vi "Autorunner.vi"() -> ()   [LabVIEW 2017, in "Fridge Software v2.1.lvlib"]
uses:
  Fridge Software v2.1.lvlib
  <vilib>/Platform/TimedLoop/XDataNode/timing_clust.ctl
  <vilib>/Platform/TimedLoop/XDataNode/nitl_modes.ctl
  <vilib>/Platform/TimedLoop/XDataNode/wakeup.ctl
  <vilib>/Utility/file.llb/Read Delimited Spreadsheet (DBL).vi
  <vilib>/Utility/file.llb/Read Delimited Spreadsheet (string).vi
  <vilib>/Utility/file.llb/Write Delimited Spreadsheet (DBL).vi
  <vilib>/platform/TimedLoop/XDataNode/XDataNode.xnode
  <instrlib>/Lake Shore 372/Lake Shore 372.lvlib
  <instrlib>/Keithley 3706/Keithley 3700 Series.lvlib
  <vilib>/Platform/TimedLoop/XDataNode/XDNodeRunTimeDep.lvlib
panel:
  in  "R(T,H) tab":enum32{"R(T)", "R(H)"}(tab)
  in  "Clear R(T) graph":bool
  in  "Autoscale R(T)":bool=TRUE caption="Autoscale"
  out "R(T) Graph":cluster{dbl[], dbl[]}(graph)
  in  "Clear H(T) graph":bool
  in  "Autoscale H(T)":bool=TRUE caption="Autoscale"
  out "R(H) Graph":cluster{dbl[], dbl[]}(graph)
  in  "Clear H(t) graph":bool
  in  "Clear T(t) graph":bool
  in  "Clear R(t) graph":bool
  in  "Autoscale H(t)":bool=TRUE caption="Autoscale"
  in  "Autoscale T(t)":bool=TRUE caption="Autoscale"
  in  "Autoscale R(t)":bool=TRUE caption="Autoscale"
  out "H(t) Graph 4":cluster{dbl[], dbl[]}(graph)
  out "T(t) Graph 3":cluster{dbl[], dbl[]}(graph)
  out "R(t) Graph":cluster{dbl[], dbl[]}(graph)
  out "Input Reading Status Query":string
  out "Elapsed time":dbl=500.0 min=50.0 step=100.0
  out "Magnetic Poles \nLive  Voltage":dbl format="%#_5g"
  in  "Measurement\nperiod":i64=500 min=100 step=100
  out "Power Reading":dbl min=0.0 max=0.01 step=1e-05 format="%^.3g"
  out "Sample Reactance":dbl min=0.0 max=63200000.0 step=1e-05 format="%.3g"
  out "Cernox Resistance":dbl min=0.0 max=63200000.0 step=1e-05 format="%.3g"
  out "Sample Resistance":dbl min=0.0 max=63200000.0 step=1e-05 format="%^.5g"
  out "Cernox Temperature":dbl min=0.0 max=1000.0 step=1e-05 format="%.4f"
  in  "Measurement":T1(tab)
  in  "Hall probe/Aux":bool
  in  "Lakeshore port":refnum<visa-resource-name>="COM6"
  in  "Cernox Channel":u16(ring)=17 caption="Cernox" items=["1"=1, "2"=2, "3"=3, "4"=4, "5"=5, "6"=6, "7"=7, "8"=8, "9"=9, "10"=10, "11"=11, "12"=12, "13"=13, "14"=14, "15"=15, "16"=16, "A"=17]
  in  "Sample Channel":u16(ring)=1 caption="Sample" items=["1"=1, "2"=2, "3"=3, "4"=4, "5"=5, "6"=6, "7"=7, "8"=8, "9"=9, "10"=10, "11"=11, "12"=12, "13"=13, "14"=14, "15"=15, "16"=16, "A (Control Input)"=17]
  in  "Switchboard port":refnum<visa-resource-name>="USB0::0x05E6::0x3706::04089883::INSTR"
  in  "Arduino port \n(for magnetic poles)":refnum<visa-resource-name>="COM3"
  out "Lakeshore Error":errorcluster
  in  "Update":bool
  out "Excitation  Ind":bool=TRUE
  out "Excitation Mode Ind":u16(ring)=1 items=["Voltage", "Current"]
  out "Excitation Range Ind":u16(ring)=19 items=["31.6 mA"=22, "10.0 mA"=21, "3.16 mA"=20, "1.00 mA"=19, "316 uA"=18, "100 uA"=17, "31.6 uA"=16, "10.0 uA"=15, "3.16 uA"=14, "1.00 uA"=13, "632 mV / 316 nA"=12, "200 mV / 100 nA"=11, "63.2 mV / 31.6 nA"=10, "20.0 mV / 10.0 nA"=9, "6.32 mV / 3.16 nA"=8, "2.00 mV / 1.00 nA"=7, "632 uV / 316 pA"=6, "200 uV / 100 pA"=5, "63.2 uV / 31.6 pA"=4, "20.0 uV / 10.0 pA"=3, "6.32 uV / 3.16 pA"=2, "2.00 uV / 1.00 pA"=1]
  out "Autorange Ind":u16(ring) items=["Autorange off", "Autorange Current", "ROX 102B Autorange"]
  out "Resistance Range Ind":u16(ring)=8 items=["63.2 MOhm"=22, "20.0 MOhm"=21, "6.32 MOhm"=20, "2.00 MOhm"=19, "632 kOhm"=18, "200 kOhm"=17, "63.2 kOhm"=16, "20.0 kOhm"=15, "6.32 kOhm"=14, "2.00 kOhm"=13, "632 Ohm"=12, "200 Ohm"=11, "63.2 Ohm"=10, "20.0 Ohm"=9, "6.32 Ohm"=8, "2.00 Ohm"=7, "632 mOhm"=6, "200 mOhm"=5, "63.2 mOhm"=4, "20.0 mOhm"=3, "6.32 mOhm"=2, "2.00 mOhm"=1]
  out "Preferred Units Ind":u16(ring)=2 items=["Kelvin"=1, "Ohms"=2]
  out "Temperature Limit Ind":dbl min=0.0 max=2999.0 step=1.0
  in  "Excitation Mode":u16(ring)=1 items=["Voltage", "Current"]
  in  "Excitation Range":u16(ring)=19 items=["31.6 mA"=22, "10.0 mA"=21, "3.16 mA"=20, "1.00 mA"=19, "316 uA"=18, "100 uA"=17, "31.6 uA"=16, "10.0 uA"=15, "3.16 uA"=14, "1.00 uA"=13, "632 mV / 316 nA"=12, "200 mV / 100 nA"=11, "63.2 mV / 31.6 nA"=10, "20.0 mV / 10.0 nA"=9, "6.32 mV / 3.16 nA"=8, "2.00 mV / 1.00 nA"=7, "632 uV / 316 pA"=6, "200 uV / 100 pA"=5, "63.2 uV / 31.6 pA"=4, "20.0 uV / 10.0 pA"=3, "6.32 uV / 3.16 pA"=2, "2.00 uV / 1.00 pA"=1]
  in  "Autorange (0: Autorange off)":u16(ring) items=["Autorange off", "Autorange Current", "ROX 102B Autorange"]
  in  "Resistance Range":u16(ring)=8 items=["63.2 MOhm"=22, "20.0 MOhm"=21, "6.32 MOhm"=20, "2.00 MOhm"=19, "632 kOhm"=18, "200 kOhm"=17, "63.2 kOhm"=16, "20.0 kOhm"=15, "6.32 kOhm"=14, "2.00 kOhm"=13, "632 Ohm"=12, "200 Ohm"=11, "63.2 Ohm"=10, "20.0 Ohm"=9, "6.32 Ohm"=8, "2.00 Ohm"=7, "632 mOhm"=6, "200 mOhm"=5, "63.2 mOhm"=4, "20.0 mOhm"=3, "6.32 mOhm"=2, "2.00 mOhm"=1]
  in  "Preferred Units (2: Ohms)":u16(ring)=2 items=["Kelvin"=1, "Ohms"=2]
  in  "Temperature Limit (0 Kelvin)":dbl min=0.0 max=2999.0 step=1.0
  in  "Excitation  (T: On)":bool=TRUE caption="On\n\nOff"
  in  "Grab settings":bool
  out "Heater Output Ind":dbl
  out "Heater Setpoint":dbl
  out "Heater Setpoint Ind":dbl
  in  "Grab Heater settings":bool
  in  "Update Heater Settings":bool
  in  "I+":i32 min=0 max=24 step=1
  in  "I-":i32 min=0 max=24 step=1
  in  "V+":i32 min=0 max=24 step=1
  in  "V-":i32 min=0 max=24 step=1
  in  "Close pins (safe)":bool caption="Close I-V pins -> Lift ground -> Lift common -> Current on"
  in  "Lift pins (safe)":bool caption="Current off -> Common closed -> Ground -> Lift I-V pins"
  in  "Channel Open/Close Array":string
  in  "Open":bool
  in  "Close":bool
  in  "Open All IV":bool
  out "Closed Channels":string
  out "Ground closed":bool
  out "Common rail \nclosed":bool
  out "Common-ground \nlink closed":bool
  in  "Append file":bool
  in  "File path":path
  in  "Save Data":bool
  in  "Aux max voltage (mV)":dbl
  in  "Aux Field Range (Oe)":dbl
  in  "Skip temperature checker":bool
  in  "Data Acquisition time\n(mins)":dbl
  in  "T Array File":path
  in  "Device/Pin Array File":path
  # "Autorunner"
  # "Created by Daniel Bromley & Alex Wright, IPF Ltd 2021"
  # "s"
  # "V"
  # "ms"
  # "W"
  # "jW"
  # "W"
  # "W"
  # "K"
  # "Lakeshore - Measurement"
  # "Channels:"
  # "Keithley - Switchboard"
  # "Hall probe"
  # "Aux"
  # "Lakeshore setting"
  # "User setting"
  # "Excitation Mode"
  # "Excitation Range"
  # "Autorange"
  # "Resistance Range"
  # "Preferred Units"
  # "Temperature Limit"
  # "Excitation"
  # "Lakeshore setting"
  # "User setting"
  # "Heater Setpoint"
  # "Heater output"
  # "IV pins"
  # "Array"
  # "Set Filename and Path"
  # "(Will be appended by Device name and temperature)"
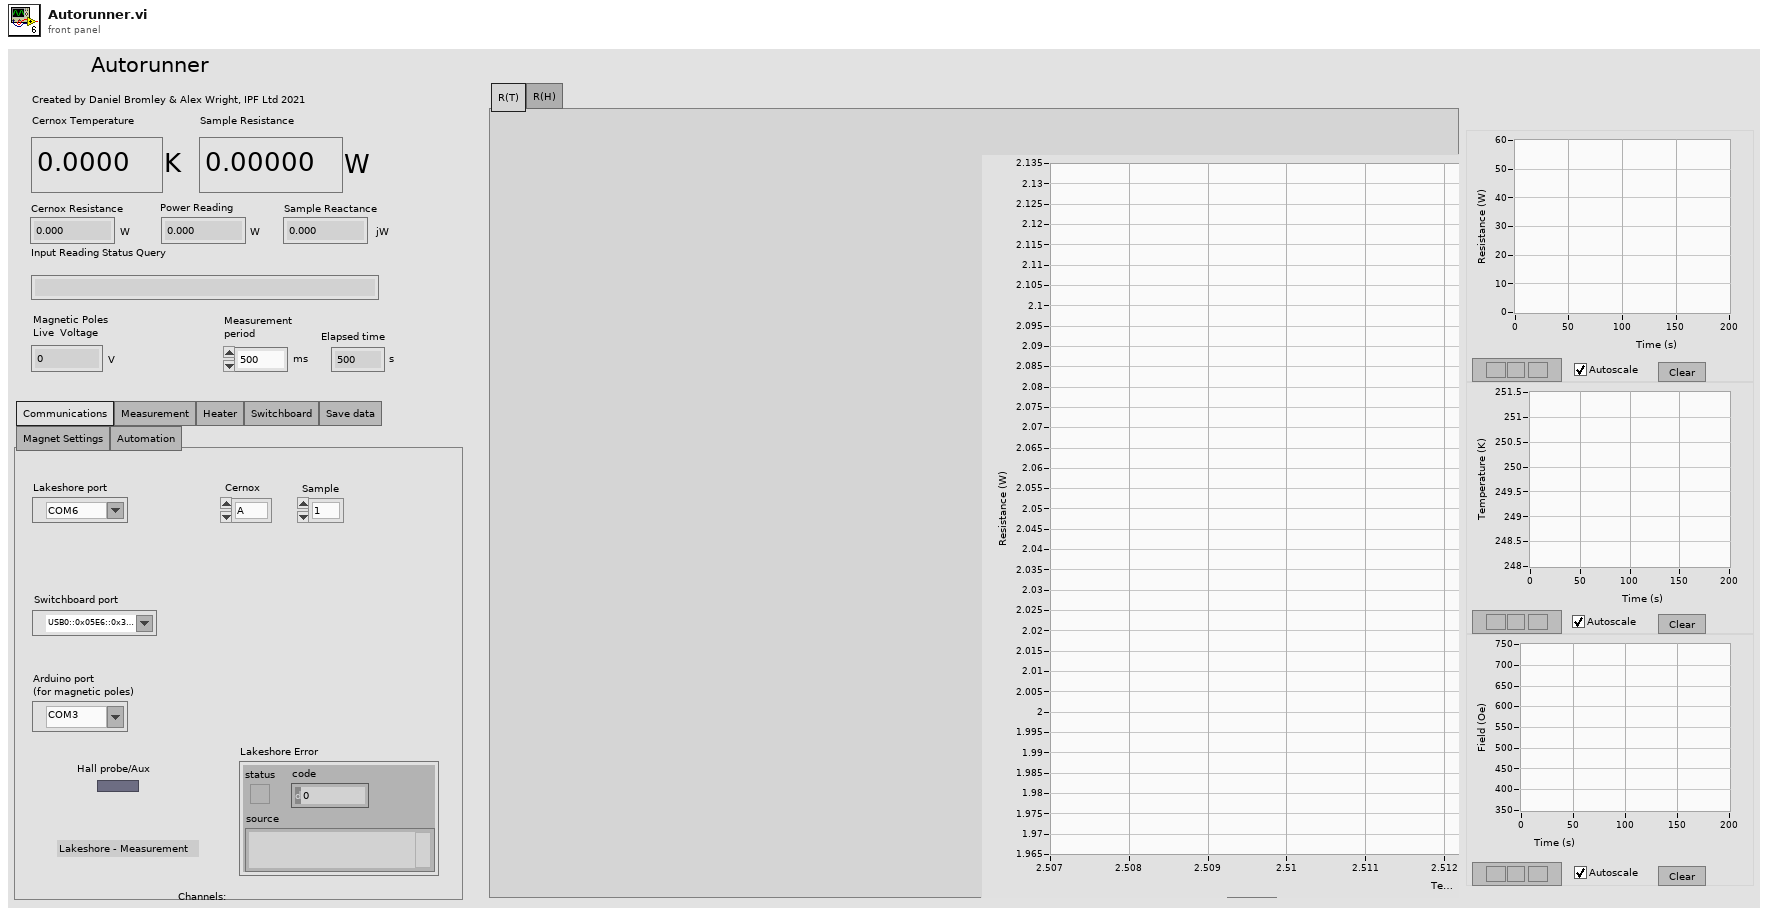
[diagram p1: front panel]
types:
  T1 = enum32{"Communications", "Measurement", "Heater", "Switchboard", "Save data", "Magnet Settings", "Automation"}
  T2 = typedef "XDNodeRunTimeDep.lvlib/timing_clust.ctl" = cluster{"Expected End [f-1]":u64, "Actual End [f-1]":u64, "Finished Late? [f-1]":bool, "Expected End [i-1]":u64, "Actual End [i-1]":u64, "Finished Late? [i-1]":bool, "Expected Start [i]":u64, "Actual Start [i]":u64, "Expected Start [f]":u64, "Actual Start [f]":u64, "Source Name":string, "Structure Name":string, "Period":i64, "Deadline":i64, "Offset":i64, "Start":i64, "Priority":i32, "Timeout":i32, "Mode":T3, "Wakeup Reason":T4, "Error":errorcluster, "Source Type":string, "Secondary Source Type":string, "Global End Time":u64, "Global Start Time":u64, "Frame Duration":u64, "Iteration Duration":u64, "Assigned CPU":i32, "I/O Scan Engine Mode":u32}
  T3 = typedef "XDNodeRunTimeDep.lvlib/nitl_modes.ctl" = enum32{"No Change", "Process missed periods, maintain original phase", "Discard missed periods, maintain original phase", "Process missed periods, ignore original phase", "Discard missed periods, ignore original phase"}
  T4 = typedef "XDNodeRunTimeDep.lvlib/wakeup.ctl" = enum32{"Normal", "Aborted", "Asynchronous wakeup", "Timing source error", "Timed loop error", "Timeout"}
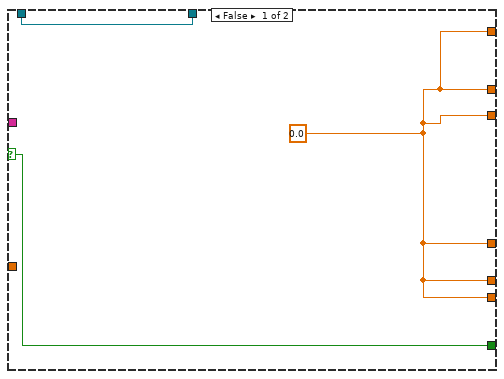
[diagram p3: hidden frame]
diagram:
  w42 = FALSE
  (unwired) TRUE
  (unwired) 11
  (unwired) TRUE
  # "Switchboard comms"
  # "Magnet Arduinio comms"
  # "Lakeshore comms"
  # "Request and read closed list from switchboard"
  # "Get closed list"
  # "Read Lakeshore settings"
  n1 = call <instrlib>:"InputChannelToString.vi"("Channel (1)"="Cernox Channel") -> ("Channel Str"=w31:string)  [unwired: 10 in]
  n2 = call <instrlib>:"InputChannelToString.vi"("Channel (1)"="Sample Channel") -> ("Channel Str"=w6:string)  [unwired: 10 in]
  n3 = call <instrlib>:"Initialize.vi"("Reset (True)"=w42, "ID Query (True)"=w42, "VISA resource name"="Lakeshore port") -> ("error out"=w34:errorcluster, "VISA resource name out"=w35:refnum<visa-resource-name>)  [unwired: 7 in]
  n4 = call "ReadLakeshoreSettings (SubVI).vi"("error in (no error)"=w34, "Channel Str"=w6, "Lakeshore port"=w35) -> ("error out"=w36:errorcluster, "Settings array out"=w4:i32[], "VISA Refnum out"=w37:refnum<visa-resource-name>)  [unwired: 4 in]
  n5 = call "ReadHeaterSettings.vi"("error in (no error)"=w36, "VISA Refnum in"=w37) -> ("error out"=w32:errorcluster, "Settings array out"=w3:dbl[], "VISA Refnum out"=w33:refnum<visa-resource-name>)  [unwired: 7 in]
  n6 = Index Array(array=w4) -> (element #1=w29:i32, element #2=w28:i32, element #3=w27:i32, element #4=w26:i32, element #5=w25:i32, element #6=w24:i32)  [unwired: 6 in]
  n7 = Index Array(array=w3) -> (element #1=→"Heater Setpoint Ind":dbl, element #2=→"Heater Output Ind":dbl)  [unwired: 2 in]
  n8 = To Unsigned Word Integer(number=w29) -> (unsigned 16bit integer=w23:u16)
  n9 = To Unsigned Word Integer(number=w28) -> (unsigned 16bit integer=w22:u16)
  n10 = To Unsigned Word Integer(number=w27) -> (unsigned 16bit integer=w21:u16)
  n11 = To Unsigned Word Integer(number=w26) -> (unsigned 16bit integer=w20:u16)
  n12 = Equal To 0?(x=w25) -> (x = 0?=w19:bool)
  n13 = To Unsigned Word Integer(number=w24) -> (unsigned 16bit integer=w18:u16)
  n14 = local write "Excitation Mode Ind"(w23) -> ()
  n15 = local write "Excitation Range Ind"(w22) -> ()
  n16 = local write "Autorange Ind"(w21) -> ()
  n17 = local write "Resistance Range Ind"(w20) -> ()
  n18 = local write "Excitation  Ind"(w19) -> ()
  n19 = local write "Preferred Units Ind"(w18) -> ()
  n20 = VISA Clear(VISA resource name="Switchboard port") -> (VISA resource name out=w10:refnum<visa-resource-name>)  [unwired: 1 in, 1 out]
  n21 = VISA Write(VISA resource name=w10, write buffer="print(channel.getclose(\"allslots\"))") -> (VISA resource name out=w16:refnum<visa-resource-name>, error out=w15:errorcluster)  [unwired: 1 in, 1 out]
  n22 = VISA Read(VISA resource name=w16, byte count=u32 1024 ("Bytes To Read (1024)"), error in (no error)=w15) -> (VISA resource name out=w17:refnum<visa-resource-name>, read buffer=w9:string, error out=w12:errorcluster)  [unwired: 1 out]
  n23 = call-poly <vilib>:"Read Delimited Spreadsheet.vi"("file path (dialog if empty)"="T Array File", "delimiter (\\t)"=",") -> ("first row"=w50:dbl[])  [unwired: 8 in, 5 out]
  n24 = call-poly <vilib>:"Read Delimited Spreadsheet.vi"("file path (dialog if empty)"="Device/Pin Array File", "delimiter (\\t)"=",") -> ("all rows"=w46:string[][])  [unwired: 8 in, 5 out]
  n25 = call "Arduino initialize (SubVI).vi"("VISA Refnum in"="Arduino port \n(for magnetic poles)") -> ("VISA Refnum out"=w30:refnum<visa-resource-name>)  [unwired: 9 in, 1 out]
  n26 = local write "Closed Channels"(w9) -> ()
  n27 = call <instrlib>:"ke37xx Error Query (Multiple).vi"("VISA resource name"=w17, "error in (no error)"=w12) -> ("VISA resource name out"=w8:refnum<visa-resource-name>, "error out"=w7:errorcluster)  [unwired: 10 in, 2 out]
  n28 = Delete From Array(array=w46, index (row)=0) -> (array with subset deleted=w45:string[][])  [unwired: 2 in, 1 out]
  n29 = Tick Count (ms)() -> (millisecond timer value=w5:u32)
  n30 = for {
    tunnel: w50 -> [w63] mode=indexing
    tunnel: w45 -> [w67]
    tunnel: w33 -> [w56]
    tunnel: w32 -> [w54]
    tunnel: w31 -> [w62]
    tunnel: w30 -> [w66]
    tunnel: w8 -> [w65]
    tunnel: w7 -> [w64]
    tunnel: w6 -> [w61]
    tunnel: w5 -> [_]
    tunnel: w4 -> [w51]
    # "Loop over temperatures"
    n31 = flat-sequence {
      tunnel: w63 -> [w77]
      tunnel: w56 -> [w74]
      tunnel: w62 -> [w76]
      tunnel: w61 -> [w78]
      tunnel: w54 -> [w73]
      tunnel: [w72] -> w60
      tunnel: [w71] -> w59
      tunnel: [w78] -> w58
      tunnel: [w76] -> w57
      tunnel: [w77] -> w52
      tunnel: w60 -> [w93]
      tunnel: w59 -> [w92]
      tunnel: w58 -> [w91]
      tunnel: w57 -> [w90]
      tunnel: [w89] -> w55
      tunnel: [w88] -> w53
      tunnel: w52 -> [w84]
      frame #0 {
        # "Set temperature and wait"
        n32 = Format Into String(format string="SETP %s %f;", "1", w77) -> (resulting string=w75:string)  [unwired: 2 in, 1 out]
        n33 = call "ReadHeaterSettings.vi"("Prepended command"=w75, "error in (no error)"=w73, "VISA Refnum in"=w74) -> ("error out"=w71:errorcluster, "Settings array out"=w70:dbl[], "VISA Refnum out"=w72:refnum<visa-resource-name>)  [unwired: 6 in]
        n34 = Index Array(array=w70) -> (element #1=w69:dbl, element #2=w68:dbl)  [unwired: 2 in]
        n35 = local write "Heater Setpoint Ind"(w69) -> ()
        n36 = local write "Heater Output Ind"(w68) -> ()
        "Heater Setpoint" <- w77
      }
      frame #1 {
        n37 = node-c288(500) -> (w83:T2)  [unwired: 1 in]
        n38 = Initialize Array(0.0, 120.0) -> (w85:dbl[])
        n39 = timed-loop {
          tunnel: w93 -> [w118]
          tunnel: w92 -> [w117]
          tunnel: w91 -> [w112]
          tunnel: w90 -> [w113]
          tunnel: [w99] -> w89
          tunnel: [w97] -> w88
          shift-right: [w106] -> _
          shift-left: w85 -> [w111]
          tunnel: [w105] -> _
          tunnel: w84 -> [w104]
          timing: w83 -> [_]
          timing-out: [_] -> w82
          stop <- w102 stop-if-true
          w114 = nan
          # "This is only to skip the T checker while writing/testing the code"
          # "Format string for buffer read"
          n40 = node-c288() -> ()  [unwired: 1 in, 1 out]
          n41 = call "QueryLakeshoreMeasurement (SubVI).vi"("error in (no error)"=w117, "Sample Channel Str"=w112, "Cernox channel string"=w113, "VISA Refnum in"=w118) -> ("error out"=w98:errorcluster, "Read output"=w115:string, "VISA Refnum out"=w100:refnum<visa-resource-name>)  [unwired: 4 in, 1 out]
          n42 = Scan From String(format string="%f%.;;%f%.;;%f%.;;%f%.;;%f%.;;%f%.;", input string=w115, default 1=w114, default 2=w114, default 3=w114, default 4=w114, default 5=w114, default 6=w114) -> (output 2=w109:dbl)  [unwired: 7 in, 3 out]
          n43 = Array Subset(array=w111, index=0, length=119) -> (w108:dbl[])
          n44 = local write "Cernox Temperature"(w109) -> ()
          n45 = Build Array (concatenate)(w109, w108) -> (w106:dbl[])
          n46 = call "ReadHeaterSettings.vi"("error in (no error)"=w98, "VISA Refnum in"=w100) -> ("error out"=w97:errorcluster, "Settings array out"=w96:dbl[], "VISA Refnum out"=w99:refnum<visa-resource-name>)  [unwired: 7 in]
          n47 = call "StableTReached (SubVI).vi"("Numeric"=w104, "Array"=w106) -> ("Boolean"=w103:bool, "mean"=w105:dbl)  [unwired: 8 in]
          n48 = Index Array(array=w96) -> (element #1=w95:dbl, element #2=w94:dbl)  [unwired: 2 in]
          n49 = Or(x=w103, y="Skip temperature checker") -> (x .or. y?=w102:bool)
          n50 = local write "Heater Setpoint Ind"(w95) -> ()
          n51 = local write "Heater Output Ind"(w94) -> ()
          n52 = node-c288() -> ()  [unwired: 1 in, 1 out]
        }
        n53 = node-c288(w82) -> ()  [unwired: 1 out]
      }
    }
    n54 = for {
      tunnel: w67 -> [w177] mode=indexing
      tunnel: w63 -> [w175]
      tunnel: w55 -> [w171]
      tunnel: w53 -> [w170]
      tunnel: w62 -> [w162]
      tunnel: w66 -> [w164]
      tunnel: w65 -> [w168]
      tunnel: w64 -> [w166]
      tunnel: w61 -> [w173]
      tunnel: w51 -> [w174]
      # "Loop over devices/pins"
      n55 = flat-sequence {
        tunnel: w174 -> [w202]
        tunnel: w173 -> [w204]
        tunnel: w175 -> [w207]
        tunnel: w177 -> [w208]
        tunnel: [w226] -> w172
        tunnel: w171 -> [w205]
        tunnel: w170 -> [w206]
        tunnel: [w212] -> w169
        tunnel: w168 -> [w212]
        tunnel: [w211] -> w167
        tunnel: w166 -> [w211]
        tunnel: [w210] -> w165
        tunnel: w164 -> [w210]
        tunnel: [w209] -> w163
        tunnel: w162 -> [w209]
        tunnel: [w195] -> w161
        tunnel: [w204] -> w160
        tunnel: [w208] -> w159
        tunnel: [w207] -> w158
        tunnel: [w183] -> w157
        tunnel: [w184] -> w156
        tunnel: w172 -> [w254]
        tunnel: w169 -> [w251]
        tunnel: w167 -> [w250]
        tunnel: w165 -> [w244]
        tunnel: w163 -> [w243]
        tunnel: w161 -> [w245]
        tunnel: w160 -> [w241]
        tunnel: w159 -> [w229]
        tunnel: w158 -> [w230]
        tunnel: w157 -> [w253]
        tunnel: w156 -> [w252]
        tunnel: [w254] -> w155
        tunnel: [w238] -> w154
        tunnel: [w237] -> w153
        tunnel: [w235] -> w152
        tunnel: [w233] -> w151
        tunnel: [w231] -> w150
        tunnel: [w244] -> w149
        tunnel: [w241] -> w148
        tunnel: [w243] -> w147
        tunnel: [w230] -> w128
        tunnel: [w229] -> w126
        tunnel: w155 -> [w307]
        tunnel: w154 -> [w328]
        tunnel: w153 -> [w327]
        tunnel: w152 -> [w324]
        tunnel: w151 -> [w321]
        tunnel: w150 -> [w308]
        tunnel: w149 -> [w319]
        tunnel: w148 -> [w322]
        tunnel: w147 -> [w323]
        tunnel: [w306] -> w146
        tunnel: [w328] -> w145
        tunnel: [w327] -> w144
        tunnel: [w324] -> w143
        tunnel: [w321] -> w142
        tunnel: [w308] -> w141
        tunnel: [w318] -> w140
        tunnel: [w322] -> w139
        tunnel: [w323] -> w138
        tunnel: w128 -> [w305]
        tunnel: [w305] -> w127
        tunnel: w126 -> [w304]
        tunnel: [w304] -> w125
        tunnel: w146 -> [w431]
        tunnel: w145 -> [w430]
        tunnel: w144 -> [w429]
        tunnel: w143 -> [w423]
        tunnel: w142 -> [w422]
        tunnel: w141 -> [w421]
        tunnel: w140 -> [w428]
        tunnel: w139 -> [w416]
        tunnel: w138 -> [w427]
        tunnel: [w431] -> w137
        tunnel: [w430] -> w136
        tunnel: [w429] -> w135
        tunnel: [w414] -> w134
        tunnel: [w413] -> w133
        tunnel: [w415] -> w132
        tunnel: [w428] -> w131
        tunnel: [w416] -> w130
        tunnel: [w427] -> w129
        tunnel: w127 -> [_]
        tunnel: w125 -> [w419]
        tunnel: [w502] -> _
        tunnel: [w501] -> _
        tunnel: [w503] -> _
        tunnel: [w498] -> _
        tunnel: [w480] -> _
        tunnel: [w479] -> _
        tunnel: [w484] -> _
        tunnel: [w483] -> _
        tunnel: [w504] -> _
        tunnel: w137 -> [w504]
        tunnel: w136 -> [w486]
        tunnel: w135 -> [w485]
        tunnel: w134 -> [w482]
        tunnel: w133 -> [w481]
        tunnel: w132 -> [w500]
        tunnel: w131 -> [w503]
        tunnel: w130 -> [w501]
        tunnel: w129 -> [w502]
        frame #0 {
          w187 = ".csv"
          # "Lakeshore comms"
          # "Switchboard comms"
          # "Magnet Arduinio comms"
          # "Switchboard comms"
          # "Magnet Arduinio comms"
          # "Lakeshore comms"
          # "Set filepath"
          # "Set current to 100 nA"
          n56 = Index Array(array=w208) -> (element=w216:string)  [unwired: 1 in]
          n57 = Format Into String(format string=", %.1f K", w207) -> (resulting string=w214:string)  [unwired: 2 in, 1 out]
          n58 = Strip Path(path="File path") -> (stripped path=w213:path, name=w188:string)
          n59 = Concatenate Strings(", ", w216, w214, w187) -> (w186:string)
          n60 = Search and Replace String(input string=w188, search string=w187, replace string=w186) -> (result string=w185:string)  [unwired: 5 in, 3 out]
          n61 = Build Path(base path=w213, name or relative path=w185) -> (appended path=w226:path)
          n62 = Index Array(array=w202) -> (element #1=w224:i32, element #3=w223:i32, element #4=w222:i32, element #5=w221:i32, element #6=w220:i32)  [unwired: 6 in, 1 out]
          n63 = Format Into String(format string="INTYPE %s,%d,%d,%d,%d,%d,%d;", w204, w224, 11, w223, w222, w221, w220) -> (resulting string=w203:string)  [unwired: 2 in, 1 out]
          n64 = call "ReadLakeshoreSettings (SubVI).vi"("Prepended command"=w203, "error in (no error)"=w206, "Channel Str"=w204, "Lakeshore port"=w205) -> ("error out"=w178:errorcluster, "Settings array out"=w195:i32[], "VISA Refnum out"=w179:refnum<visa-resource-name>)  [unwired: 3 in]
          n65 = Index Array(array=w195) -> (element #1=w201:i32, element #2=w200:i32, element #3=w199:i32, element #4=w198:i32, element #5=w197:i32, element #6=w196:i32)  [unwired: 6 in]
          n66 = call "ReadHeaterSettings.vi"("error in (no error)"=w178, "VISA Refnum in"=w179) -> ("error out"=w184:errorcluster, "Settings array out"=w182:dbl[], "VISA Refnum out"=w183:refnum<visa-resource-name>)  [unwired: 7 in]
          n67 = To Unsigned Word Integer(number=w201) -> (unsigned 16bit integer=w194:u16)
          n68 = To Unsigned Word Integer(number=w200) -> (unsigned 16bit integer=w193:u16)
          n69 = To Unsigned Word Integer(number=w199) -> (unsigned 16bit integer=w192:u16)
          n70 = To Unsigned Word Integer(number=w198) -> (unsigned 16bit integer=w190:u16)
          n71 = Equal To 0?(x=w197) -> (x = 0?=w191:bool)
          n72 = To Unsigned Word Integer(number=w196) -> (unsigned 16bit integer=w189:u16)
          n73 = Index Array(array=w182) -> (element #1=w181:dbl, element #2=w180:dbl)  [unwired: 2 in]
          n74 = local write "Excitation Mode Ind"(w194) -> ()
          n75 = local write "Excitation Range Ind"(w193) -> ()
          n76 = local write "Autorange Ind"(w192) -> ()
          n77 = local write "Resistance Range Ind"(w190) -> ()
          n78 = local write "Excitation  Ind"(w191) -> ()
          n79 = local write "Preferred Units Ind"(w189) -> ()
          n80 = local write "Heater Setpoint Ind"(w181) -> ()
          n81 = local write "Heater Output Ind"(w180) -> ()
        }
        frame #1 {
          n82 = Array Subset(array=w229, index=1, length=4) -> (w247:string[])
          n83 = Decimal String To Number(string=w247) -> (number=w246:i32[])  [unwired: 2 in, 1 out]
          n84 = call "SafeClosePins (SubVI).vi"("Lakeshore VISA Refnum in"=w253, "Settings array in"=w245, "Lakeshore error in (no error)"=w252, "Channel Str"=w241, "Switchboard VISA resource name in"=w251, "Switchboard error in"=w250, "Pin array in"=w246) -> ("Settings array out"=w232:i32[], "Lakeshore VISA Refnum out 2"=w236:refnum<visa-resource-name>, "Lakeshore error out 2"=w234:errorcluster, "Switchboard VISA Refnum out"=w238:refnum<visa-resource-name>, "Switchboard error out"=w237:errorcluster)  [unwired: 4 in]
          n85 = Wait (ms)(milliseconds to wait=5000) -> ()  [unwired: 1 out]
          n86 = node-c288(5000) -> (w240:T2)  [unwired: 1 in]
          n87 = timed-loop {
            tunnel: w232 -> [w290]
            tunnel: w241 -> [w287]
            tunnel: w236 -> [w289]
            tunnel: w234 -> [w288]
            shift-right: [w272] -> _
            shift-left: 11 -> [w270]
            tunnel: [w259] -> w235
            tunnel: [w258] -> w233
            timing: w240 -> [_]
            timing-out: [_] -> w239
            tunnel: [w274] -> w231
            tunnel: w229 -> [w268]
            stop <- w271 stop-if-true
            # "Current on \n(Shunt off)"
            # "Ramp current up to selected current, waiting 5 seconds between ramps"
            # "Generate settings command string"
            n88 = node-c288() -> ()  [unwired: 1 in, 1 out]
            n89 = Decimal String To Number(string=w268) -> (number=w267:i32[])  [unwired: 2 in, 1 out]
            n90 = Add(x=2, y=w270) -> (x+y=w262:i32)
            n91 = Index Array(array=w267, index #1=5, index #2=6) -> (element #1=w263:i32, element #2=w265:i32)
            n92 = Greater Or Equal?(x=w262, y=w263) -> (x >= y?=w271:bool)
            n93 = Index Array(array=w290) -> (element #1=w294:i32, element #3=w293:i32, element #6=w292:i32)  [unwired: 6 in, 3 out]
            n94 = Select(t=w263, s=w271, f=w262) -> (s? t:f=w272:i32)
            n95 = Format Into String(format string="INTYPE %s,%d,%d,%d,%d,%d,%d;", w287, w294, w272, w293, w265, 0, w292) -> (resulting string=w291:string)  [unwired: 2 in, 1 out]
            n96 = call "ReadLakeshoreSettings (SubVI).vi"("Prepended command"=w291, "error in (no error)"=w288, "Channel Str"=w287, "Lakeshore port"=w289) -> ("error out"=w261:errorcluster, "Settings array out"=w274:i32[], "VISA Refnum out"=w260:refnum<visa-resource-name>)  [unwired: 3 in]
            n97 = Index Array(array=w274) -> (element #1=w286:i32, element #2=w285:i32, element #3=w284:i32, element #4=w283:i32, element #5=w282:i32, element #6=w281:i32)  [unwired: 6 in]
            n98 = call "ReadHeaterSettings.vi"("error in (no error)"=w261, "VISA Refnum in"=w260) -> ("error out"=w258:errorcluster, "Settings array out"=w257:dbl[], "VISA Refnum out"=w259:refnum<visa-resource-name>)  [unwired: 7 in]
            n99 = To Unsigned Word Integer(number=w286) -> (unsigned 16bit integer=w280:u16)
            n100 = To Unsigned Word Integer(number=w285) -> (unsigned 16bit integer=w279:u16)
            n101 = To Unsigned Word Integer(number=w284) -> (unsigned 16bit integer=w278:u16)
            n102 = To Unsigned Word Integer(number=w283) -> (unsigned 16bit integer=w277:u16)
            n103 = Equal To 0?(x=w282) -> (x = 0?=w276:bool)
            n104 = To Unsigned Word Integer(number=w281) -> (unsigned 16bit integer=w275:u16)
            n105 = local write "Excitation Mode Ind"(w280) -> ()
            n106 = local write "Excitation Range Ind"(w279) -> ()
            n107 = local write "Autorange Ind"(w278) -> ()
            n108 = local write "Resistance Range Ind"(w277) -> ()
            n109 = local write "Excitation  Ind"(w276) -> ()
            n110 = local write "Preferred Units Ind"(w275) -> ()
            n111 = Index Array(array=w257) -> (element #1=w256:dbl, element #2=w255:dbl)  [unwired: 2 in]
            n112 = local write "Heater Setpoint Ind"(w256) -> ()
            n113 = local write "Heater Output Ind"(w255) -> ()
            n114 = node-c288() -> ()  [unwired: 1 in, 1 out]
          }
          n115 = node-c288(w239) -> ()  [unwired: 1 out]
        }
        frame #2 {
          # "Graph indices array"
          # "Graph data array"
          n116 = call "Write header (SubVI).vi"("Settings array in"=w308, "Append? Out"=TRUE, "Path in"=w307) -> ("error out"=w302:errorcluster, "Path out"=w309:path)  [unwired: 7 in]
          n117 = Initialize Array(0.0, 0, 6) -> (w312:dbl[][])
          n118 = Initialize Array(0.0, 5) -> (w311:dbl[])
          n119 = Tick Count (ms)() -> (millisecond timer value=w320:u32)
          n120 = node-c288("Measurement\nperiod") -> (w326:T2)  [unwired: 3 in]
          n121 = timed-loop {
            timing: w326 -> [_]
            timing-out: [_] -> w325
            tunnel: w324 -> [w382]
            tunnel: w323 -> [w381]
            tunnel: w322 -> [w380]
            tunnel: w321 -> [w379]
            tunnel: [w373] -> _
            tunnel: w320 -> [w373]
            tunnel: w319 -> [w372]
            tunnel: [w371] -> w318
            shift-right: [w354] -> _
            shift-left: w312 -> [w363]
            shift-right: [w355] -> _
            shift-left: w311 -> [w356]
            tunnel: w309 -> [w338]
            tunnel: w308 -> [w336]
            tunnel: [w335] -> w306
            tunnel: w304 -> [w332]
            tunnel: [w330] -> _
            tunnel: w302 -> [w329]
            stop <- w348 stop-if-true
            # "Only append measurement values if we've managed to measure"
            n122 = node-c288() -> ()  [unwired: 1 in, 1 out]
            n123 = Tick Count (ms)() -> (millisecond timer value=w374:u32)
            n124 = Subtract(x=w374, y=w373) -> (x-y=w376:u32)
            n125 = Divide(x=w376, y=1000) -> (x/y=w347:dbl)
            n126 = call "QueryLakeshoreMeasurement (SubVI).vi"("error in (no error)"=w379, "Sample Channel Str"=w380, "Cernox channel string"=w381, "VISA Refnum in"=w382) -> ("Read output"=w377:string, "Boolean"=w378:bool)  [unwired: 4 in, 2 out]
            n127 = case shown="True" w378 {
              selector: w378 -> [w387 w390]
              tunnel: w377 -> [_ w403]
              tunnel: w347 -> [_ w396]
              tunnel: w372 -> [w389 w401]
              tunnel: [w389 w400] -> w371
              tunnel: [w388 w396] -> w370
              tunnel: [w388 w395] -> w369
              tunnel: [w388 w394] -> w368
              tunnel: [w388 w393] -> w367
              tunnel: [w388 w392] -> w366
              tunnel: [w388 w391] -> w365
              tunnel: [w387 w390] -> w364
              frame False {
                w388 = 0.0
              }
              frame True {
                w405 = nan
                # "Format string for buffer read"
                n128 = call "MagnetArduinoVoltageReader.vi"("Aux Field Range (Oe)"="Aux Field Range (Oe)", "Aux max voltage (mV)"="Aux max voltage (mV)", "Hall probe/Aux"="Hall probe/Aux", "VISA Refnum in"=w401) -> ("Numeric"=w393:dbl, "VISA Refnum out"=w400:refnum<visa-resource-name>)  [unwired: 5 in, 1 out]
                "Magnetic Poles \nLive  Voltage" <- w393
                n129 = Scan From String(format string="%f%.;;%f%.;;%f%.;;%f%.;;%f%.;;%f%.;", input string=w403, default 1=w405, default 2=w405, default 3=w405, default 4=w405, default 5=w405, default 6=w405) -> (output 1=w395:dbl, output 2=w394:dbl, output 3=→"Power Reading":dbl, output 4=w392:dbl, output 5=w391:dbl, output 6=w404:dbl)  [unwired: 2 in, 3 out]
                "Cernox Resistance" <- w395
                "Cernox Temperature" <- w394
                "Sample Resistance" <- w392
                "Sample Reactance" <- w391
                n130 = call "StatusQueryParser.vi"("Numeric"=w404) -> ()  [unwired: 10 in, 1 out]
                "Elapsed time" <- w396
              }
            }
            n131 = Build Array(w370, w369, w368, w367, w366, w365) -> (w337:dbl[])
            n132 = call "ParseLakeshoreSettings (SubVI).vi"("Settings array in"=w336) -> ("Current excitation (A)"=w339:dbl)  [unwired: 1 out]
            n133 = case shown="True" w364 {
              tunnel: w337 -> [_ w385]
              tunnel: [w383 w386] -> w354
              tunnel: w363 -> [w383 w384]
              frame False {
              }
              frame True {
                n134 = Build Array (concatenate)(w384, w385) -> (w386:dbl[][])
              }
            }
            n135 = Insert Into Array(array=w337, index=3, new element=w339) -> (w340:dbl[])
            n136 = Decimal String To Number(string=w332) -> (number=w334:i32[])  [unwired: 2 in, 1 out]
            n137 = Index Array(array=w334, index=7) -> (element=w331:i32)
            n138 = call-poly <vilib>:"Write Delimited Spreadsheet.vi"("file path (dialog if empty)"=w338, "format (%.3f)"="%e", "1D data"=w340, "append to file? (new file:F)"=TRUE, "error in (no error)"=w329, "delimiter (\\t)"=", ") -> ("new file path (Not A Path if cancelled)"=w335:path, "error out"=w330:errorcluster)  [unwired: 8 in]
            n139 = Build Array("Clear R(T) graph", "Clear H(T) graph", "Clear R(t) graph", "Clear T(t) graph", "Clear H(t) graph") -> (w357:bool[])
            n140 = call "Graph handler (SubVI).vi"("Data in"=w354, "Graph indices in"=w356, "Clear graph Array"=w357) -> ("Graph indices out"=w355:dbl[], "R(T) Graph"=→"R(T) Graph":cluster{dbl[], dbl[]}, "R(H) Graph"=→"R(H) Graph":cluster{dbl[], dbl[]}, "R(t) Graph"=→"R(t) Graph":cluster{dbl[], dbl[]}, "T(t) Graph 3"=→"T(t) Graph 3":cluster{dbl[], dbl[]}, "H(t) Graph 4"=→"H(t) Graph 4":cluster{dbl[], dbl[]})  [unwired: 7 in]
            n141 = Divide(x=w347, y=60) -> (x/y=w345:dbl)
            n142 = node-c288() -> ()  [unwired: 1 in, 1 out]
            n143 = Greater Or Equal?(x=w345, y=w331) -> (x >= y?=w348:bool)
          }
          n144 = node-c288(w325) -> ()  [unwired: 1 out]
        }
        frame #3 {
          n145 = Decimal String To Number(string=w419) -> (number=w420:i32[])  [unwired: 2 in, 1 out]
          n146 = node-c288(5000) -> (w426:T2)  [unwired: 3 in]
          n147 = Index Array(array=w420, index=5) -> (element=w417:i32)
          n148 = timed-loop {
            timing: w426 -> [_]
            timing-out: [_] -> w425
            tunnel: w421 -> [w459]
            tunnel: w416 -> [w458]
            tunnel: w423 -> [w457]
            tunnel: [w438] -> w414
            tunnel: w422 -> [w456]
            tunnel: [w436] -> w413
            tunnel: w416 -> [w455]
            tunnel: [w454] -> w415
            shift-right: [w447] -> _
            shift-left: w417 -> [w442]
            stop <- w446 stop-if-true
            w440 = 11
            # "Ramp current down to 100 nA, waiting 5 seconds between ramps.\nTurn off current once current is less than 100 nA"
            n149 = node-c288() -> ()  [unwired: 1 in, 1 out]
            n150 = Subtract(x=w442, y=2) -> (x-y=w439:i32)
            n151 = Less?(x=w439, y=w440) -> (x < y?=w446:bool)
            n152 = Index Array(array=w459) -> (element #1=w470:i32, element #3=w469:i32, element #4=w468:i32, element #5=w445:i32, element #6=w467:i32)  [unwired: 6 in, 1 out]
            n153 = Select(t=w440, s=w446, f=w439) -> (s? t:f=w447:i32)
            n154 = Select(t=1, s=w446, f=w445) -> (s? t:f=w443:i32)
            n155 = Format Into String(format string="INTYPE %s,%d,%d,%d,%d,%d,%d;", w458, w470, w447, w469, w468, w443, w467) -> (resulting string=w466:string)  [unwired: 2 in, 1 out]
            n156 = call "ReadLakeshoreSettings (SubVI).vi"("Prepended command"=w466, "error in (no error)"=w456, "Channel Str"=w455, "Lakeshore port"=w457) -> ("error out"=w437:errorcluster, "Settings array out"=w454:i32[], "VISA Refnum out"=w434:refnum<visa-resource-name>)  [unwired: 3 in]
            n157 = call "ReadHeaterSettings.vi"("error in (no error)"=w437, "VISA Refnum in"=w434) -> ("error out"=w436:errorcluster, "Settings array out"=w435:dbl[], "VISA Refnum out"=w438:refnum<visa-resource-name>)  [unwired: 7 in]
            n158 = Index Array(array=w454) -> (element #1=w465:i32, element #2=w464:i32, element #3=w463:i32, element #4=w462:i32, element #5=w461:i32, element #6=w460:i32)  [unwired: 6 in]
            n159 = To Unsigned Word Integer(number=w465) -> (unsigned 16bit integer=w453:u16)
            n160 = To Unsigned Word Integer(number=w464) -> (unsigned 16bit integer=w452:u16)
            n161 = To Unsigned Word Integer(number=w463) -> (unsigned 16bit integer=w451:u16)
            n162 = To Unsigned Word Integer(number=w462) -> (unsigned 16bit integer=w450:u16)
            n163 = Equal To 0?(x=w461) -> (x = 0?=w449:bool)
            n164 = To Unsigned Word Integer(number=w460) -> (unsigned 16bit integer=w448:u16)
            n165 = Index Array(array=w435) -> (element #1=w433:dbl, element #2=w432:dbl)  [unwired: 2 in]
            n166 = local write "Excitation Mode Ind"(w453) -> ()
            n167 = local write "Excitation Range Ind"(w452) -> ()
            n168 = local write "Autorange Ind"(w451) -> ()
            n169 = local write "Resistance Range Ind"(w450) -> ()
            n170 = local write "Excitation  Ind"(w449) -> ()
            n171 = local write "Preferred Units Ind"(w448) -> ()
            n172 = local write "Heater Setpoint Ind"(w433) -> ()
            n173 = local write "Heater Output Ind"(w432) -> ()
            n174 = node-c288() -> ()  [unwired: 1 in, 1 out]
          }
          n175 = node-c288(w425) -> ()  [unwired: 1 out]
        }
        frame #4 {
          n176 = call "SafeOpenPins (SubVI).vi"("LakeshoreVISA Refnum in"=w482, "Settings array in"=w500, "error in (no error)"=w481, "Channel Str"=w501, "Switchboard VISA Refnum in"=w486, "Switchboard error in"=w485) -> ("Settings array out"=w498:i32[], "VISA Refnum out"=w479:refnum<visa-resource-name>, "error out"=w480:errorcluster, "VISA resource name out"=w483:refnum<visa-resource-name>, "Switchboard error out"=w484:errorcluster)  [unwired: 5 in]
          n177 = Index Array(array=w498) -> (element #1=w497:i32, element #2=w496:i32, element #3=w494:i32, element #4=w491:i32, element #5=w492:i32, element #6=w487:i32)  [unwired: 6 in]
          n178 = To Unsigned Word Integer(number=w497) -> (unsigned 16bit integer=w499:u16)
          n179 = To Unsigned Word Integer(number=w496) -> (unsigned 16bit integer=w495:u16)
          n180 = To Unsigned Word Integer(number=w494) -> (unsigned 16bit integer=w493:u16)
          n181 = To Unsigned Word Integer(number=w491) -> (unsigned 16bit integer=w490:u16)
          n182 = Equal To 0?(x=w492) -> (x = 0?=w489:bool)
          n183 = To Unsigned Word Integer(number=w487) -> (unsigned 16bit integer=w488:u16)
          n184 = local write "Excitation Mode Ind"(w499) -> ()
          n185 = local write "Excitation Range Ind"(w495) -> ()
          n186 = local write "Autorange Ind"(w493) -> ()
          n187 = local write "Resistance Range Ind"(w490) -> ()
          n188 = local write "Excitation  Ind"(w489) -> ()
          n189 = local write "Preferred Units Ind"(w488) -> ()
          n190 = Wait (ms)(milliseconds to wait=5000) -> ()  [unwired: 1 out]
        }
      }
      n191 = Wait (ms)(milliseconds to wait=500) -> ()  [unwired: 1 out]
    }
  }
